vi "Create Child Service Class.vi"(7 "RPC Method Parameters":T1[](array[typedef]), 8 "error in (no error)":errorcluster, 10 "Service base class in":refnum<vi>, 11 "Server Library in":refnum<vi>) -> (0 "error IO":errorcluster, 1 "Service Impl class out":refnum<vi>, 2 "Service base class out":refnum<vi>, 3 "Server Library out":refnum<vi>)   [LabVIEW 2019, in "gRPC Template Creation Utility.lvlib"]
uses:
  gRPC Template Creation Utility.lvlib
  TypeDefs/RPC Method Parameters.ctl
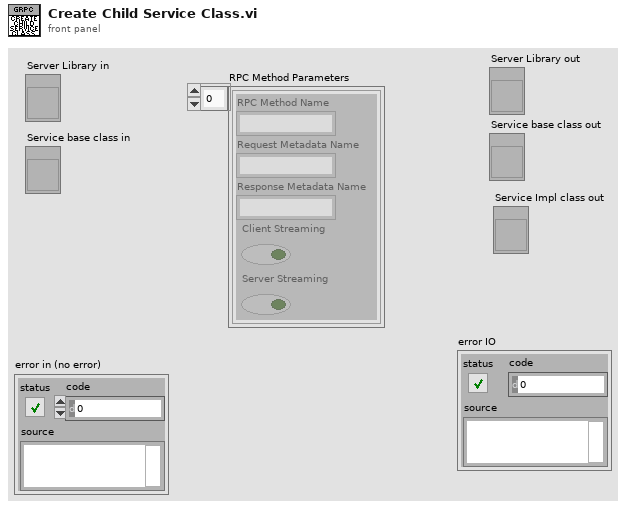
[diagram p1: front panel]
types:
  T1 = typedef "gRPC Template Creation Utility.lvlib/RPC Method Parameters.ctl" = cluster{"RPC Method Name":string, "Request Metadata Name":string, "Response Metadata Name":string, "Client Streaming":bool, "Server Streaming":bool}
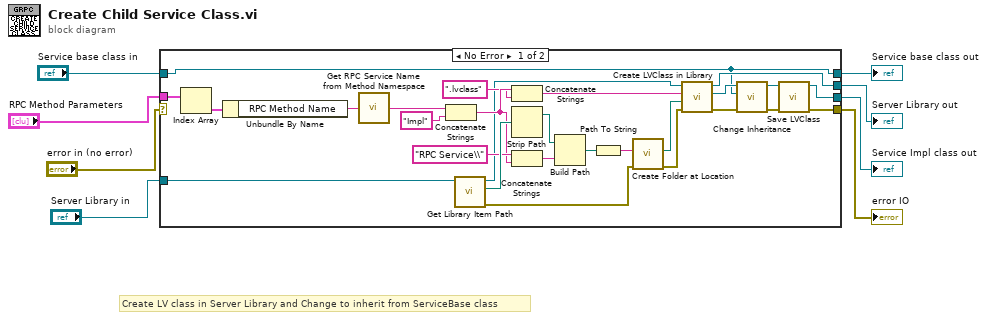
[diagram p0: block diagram]
diagram:
  # "Create LV class in Server Library and Change to inherit from ServiceBase class"
  n1 = case shown="No Error" "error in (no error)" {
    selector: "error in (no error)" -> [_ w38]
    tunnel: "RPC Method Parameters" -> [w17 _]
    tunnel: "Server Library in" -> [w14 w37]
    tunnel: [w13 _] -> w1
    tunnel: [w12 w38] -> w3
    tunnel: [w10 w37] -> w5
    tunnel: "Service base class in" -> [w9 w36]
    tunnel: [w9 w36] -> w2
    frame No Error {
      n2 = Index Array(array=w17) -> (element=w16:T1)  [unwired: 1 in]
      n3 = Unbundle By Name(w16) -> ("RPC Method Name"=w15:string)
      n4 = call "Get RPC Service Name from Method Namespace.vi"("RPC Method Name"=w15) -> ("RPC Service Name"=w28:string)
      n5 = Concatenate Strings(w28, "Impl" ("string")) -> (w24:string)
      n6 = call "Get Library Item Path.vi"("Library"=w14) -> ("error out"=w31:errorcluster, "Path"=w35:path, "Library"=w11:refnum<vi>)  [unwired: 8 in]
      n7 = Concatenate Strings(w24, ".lvclass" ("string")) -> (w22:string)
      n8 = Strip Path(path=w35) -> (stripped path=w34:path)  [unwired: 1 out]
      n9 = Concatenate Strings("RPC Service\\" ("Path"), w24) -> (w25:string)
      n10 = Build Path(base path=w34, name or relative path=w25) -> (appended path=w33:path)
      n11 = Path To String(path=w33) -> (string=w32:string)
      n12 = call "Create Folder at Location.vi"("Error In"=w31, "Path"=w32) -> ("Error Out"=w30:errorcluster, "Full path out"=w29:path)  [unwired: 7 in, 1 out]
      n13 = call "Create LVClass in Library.vi"("error in"=w30, "new class folder"=w29, "new class file name"=w22, "library reference in"=w11) -> ("error out"=w20:errorcluster, "class reference"=w21:refnum<vi>, "library reference out"=w10:refnum<vi>)  [unwired: 5 in]
      n14 = call "Change Inheritance.vi"("error in (no error)"=w20, "Parent Class"=w9, "LV Class Ref in"=w21) -> ("error out"=w18:errorcluster, "LV Class ref out"=w19:refnum<vi>)  [unwired: 7 in]
      n15 = call "Save LVClass.vi"("error in (no error)"=w18, "LVClassLibrary in"=w19) -> ("error out"=w12:errorcluster, "LVClassLibrary out"=w13:refnum<vi>)  [unwired: 8 in]
    }
    frame Error {
    }
  }
  "Server Library out" <- w5
  "error IO" <- w3
  "Service base class out" <- w2
  "Service Impl class out" <- w1
